vi "Configuration Keys.vi"(8 "error in":errorcluster, 11 "34980A in":refnum<class "34980A.lvclass">) -> (0 "error out":errorcluster, 2 "Required Keys":string[](array[string]), 3 "34980A out":refnum<class "34980A.lvclass">)   [LabVIEW 2019, in "34980A.lvlib" / "34980A.lvclass"]
uses:
  Library/34980A.lvclass
  Custom Controls/Configuration Keys.ctl
  builds/Instruments/MLTFNC.lvlibp/Library/MLTFNC.lvclass
panel:
  in  "Configuration Keys":T1
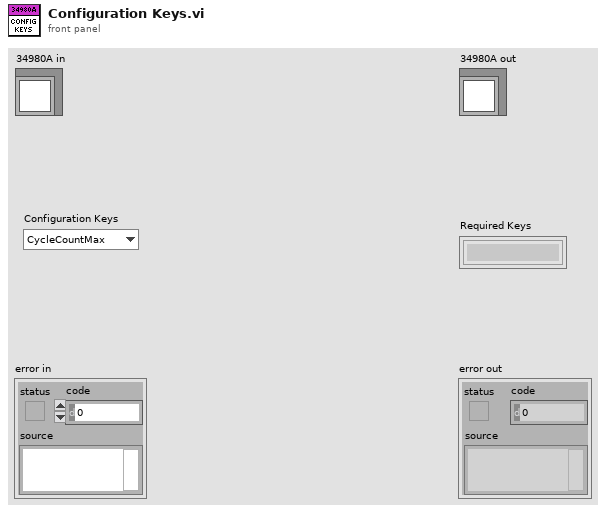
[diagram p1: front panel]
types:
  T1 = typedef "34980A.lvlib/34980A.lvclass/Configuration Keys.ctl" = enum16{"CycleCountMax"}
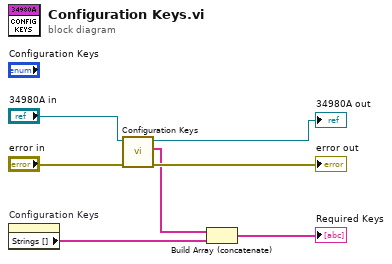
[diagram p0: block diagram]
diagram:
  n1 = property on="Configuration Keys" class="Enum (strict)"() -> ("Strings []"=w3:string[])  [unwired: 2 in, 2 out]
  n2 = call-parent "Configuration Keys.vi"("error in"="error in", "MLTFNC in"="34980A in") -> ("error out"=→"error out":errorcluster, "Required Keys"=w2:string[], "MLTFNC out"=→"34980A out":refnum<class "34980A.lvclass">)  [unwired: 7 in]
  n3 = Build Array (concatenate)(w2, w3) -> (→"Required Keys":string[])
